vi "Dpc Stream Write.vi"(0 "hif":u32, 1 "ptrid":u16, 5 "rgbData":string, 7 "cbData":i32, 9 "perc":i32, 11 "error in (no error)":errorcluster) -> (3 "ptrid out":u16, 4 "hif out":u32, 6 "rgbData out":string, 8 "function return":i32, 10 "perc out":i32, 15 "error out":errorcluster)   [LabVIEW 2011, in "LVH-Adept.lvlib" / "DPCUTIL.lvlib"]
doc: "DPCAPI BOOL DpcStreamWrite(HANDLE hif, BYTE * rgbData, INT32 cbData, ERC * perc, TRID * ptrid);"
uses:
  DPCUTIL.lvlib
  Resources/dpcutil.dll
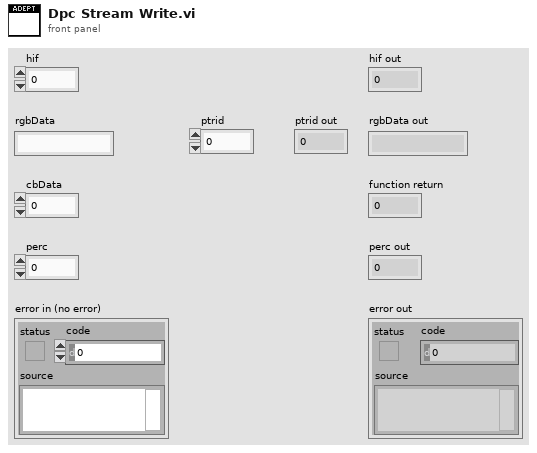
[diagram p1: front panel]
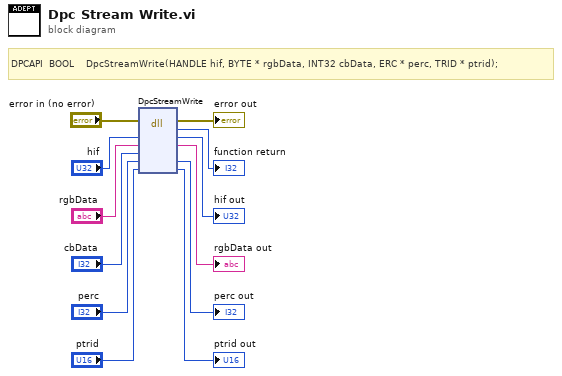
[diagram p0: block diagram]
diagram:
  # "DPCAPI  BOOL    DpcStreamWrite(HANDLE hif, BYTE * rgbData, INT32 cbData, ERC * perc, TRID * ptrid);"
  n1 = dll-call lib="C:/github/labviewhacker/LVH-Adept/LabVIEW/vi.lib/LabVIEW Hacker/Adept/Private/Resources/dpcutil.*" fn="DpcStreamWrite"(error in="error in (no error)", "hif"="hif", "rgbData"="rgbData", "cbData"="cbData", "perc"="perc", "ptrid"="ptrid") -> (error out=→"error out":errorcluster, →"function return":i32, "hif"=→"hif out":u32, "rgbData"=→"rgbData out":string, "perc"=→"perc out":i32, "ptrid"=→"ptrid out":u16)  [unwired: 3 in, 1 out]
